vi "U32ToBinary.vi"(8 "error in":errorcluster, 9 "pixmap":u32[](array[numeric]), 11 "path to pixmap.bin":path) -> (0 "error out":errorcluster)   [LabVIEW 2022 SP3]
doc: "This VI converts an U32 array to binary and saves it at a specific path\n\nIt first creates/replaces the file, second write in and finally closes it.\n\nIt uses 2 parameters :\n- The endianess\n- Whether or not it creates or replaces the file\n\nInputs :\n- The path to pixmap.bin (existant or not)\n- The pixmap (U32)\n- Error in\n\nOutputs :\n- Error out"
panel:
  in  "byte order":T1(ring)=enum."little-endian"
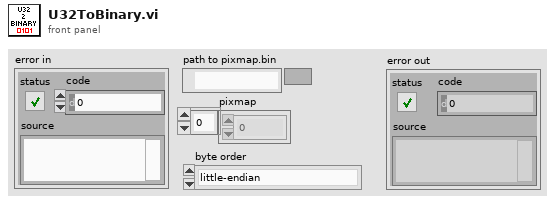
[diagram p1: front panel]
types:
  T1 = enum16{"big-endian, network order", "native, host order", "little-endian"}
  T2 = enum16{"open", "replace", "create", "open or create", "replace or create", "replace or create with confirmation"}
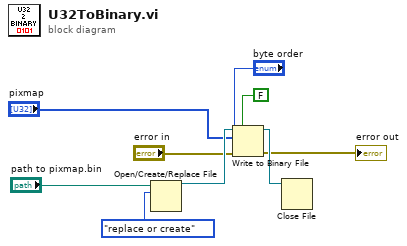
[diagram p0: block diagram]
diagram:
  n1 = Open/Create/Replace File ("Create File")(file path (use dialog)="path to pixmap.bin", operation (0:open)=T2."replace or create") -> (refnum out=w7:refnum<file>)  [unwired: 4 in, 2 out]
  n2 = Write to Binary File(file (use dialog)=w7, data="pixmap", error in="error in", 5:FALSE, 9:"byte order") -> (refnum out=w5:refnum<file>, error out=→"error out":errorcluster)  [unwired: 1 in, 1 out]
  n3 = Close File(refnum=w5) -> ()  [unwired: 1 in, 2 out]
